vi "Read Serial Configs.vi"(8 "error in (no error)":errorcluster, 10 "Item Ref in":T2 format="%.0x", 11 "Refnum in":T1) -> (0 "error out":errorcluster, 2 "Item Ref out":T2 format="%.0x", 3 "Refnum out":T1)   [LabVIEW 2015, in "Modbus Master System Explorer.lvlib"]
uses:
  Modbus Master System Explorer.lvlib
  <vilib>/Utility/config.llb/Config Data RefNum.ctl
  <vilib>/NI Veristand/Custom Device API/Custom Device Item Ref.ctl
  Shared/Controls/Flow Control.ctl
  Shared/Controls/Serial Type.ctl
  Shared/Controls/Parity.ctl
  <vilib>/Utility/config.llb/Read Key (String).vi
  <vilib>/Utility/config.llb/Read Key (U32).vi
  <vilib>/Utility/config.llb/NI_LVConfig.lvlib
  Shared/Modbus Master Shared.lvlib
  <vilib>/NI VeriStand/Custom Device API/Custom Device API.lvlib
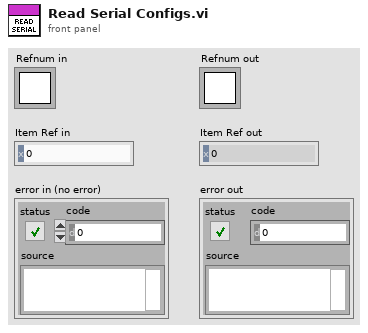
[diagram p1: front panel]
types:
  T1 = typedef "NI_LVConfig.lvlib/Config Data RefNum.ctl" = refnum<k1>
  T2 = typedef "Custom Device API.lvlib/Custom Device Item Ref.ctl" = u64
  T3 = typedef "Modbus Master Shared.lvlib/Serial Type.ctl" = enum16{"RTU", "ASCII"}
  T4 = typedef "Modbus Master Shared.lvlib/Parity.ctl" = u16
  T5 = typedef "Modbus Master Shared.lvlib/Flow Control.ctl" = u16
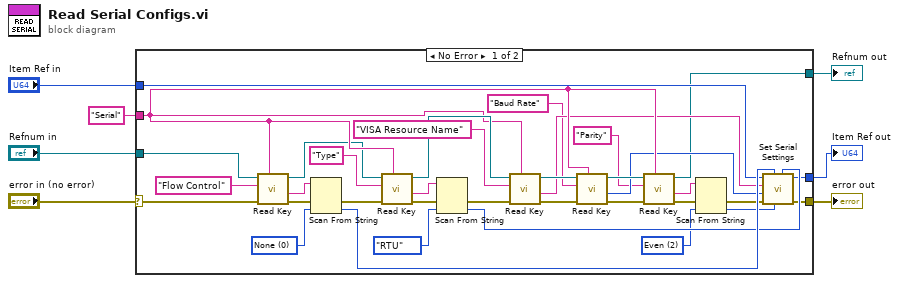
[diagram p0: block diagram]
diagram:
  n1 = case shown="No Error" "error in (no error)" {
    selector: "error in (no error)" -> [w36 w44]
    tunnel: "Refnum in" -> [w42 w43]
    tunnel: "Serial" ("section") -> [w40 _]
    tunnel: [w11 w44] -> w4
    tunnel: [w10 w45] -> w3
    tunnel: "Item Ref in" -> [w9 w45]
    tunnel: [w8 w43] -> w1
    frame No Error {
      w16 = T4 2 items=["None", "Odd", "Even", "Mark", "Space"] ("parity (even)")
      w32 = T5 0 items=["None", "XON/XOFF", "RTS/CTS", "XON/XOFF & RTS/CTS", "DTR/DSR", "XON/XOFF & DTR/DSR"] ("flow control (none)")
      n2 = call-poly <vilib>:"Read Key.vi"("section"=w40, "error in (no error)"=w36, "key"="Flow Control", "refnum"=w42) -> ("error out"=w29:errorcluster, "value"=w31:string, "refnum out"=w37:T1)  [unwired: 4 in, 1 out]
      n3 = Scan From String(input string=w31, error in=w29, default 1=w32) -> (error out=w28:errorcluster, output 1=w30:T5)  [unwired: 2 in, 2 out]
      n4 = call-poly <vilib>:"Read Key.vi"("section"=w40, "error in (no error)"=w28, "key"="Type", "refnum"=w37) -> ("error out"=w23:errorcluster, "value"=w27:string, "refnum out"=w41:T1)  [unwired: 4 in, 1 out]
      n5 = Scan From String(input string=w27, error in=w23, default 1=Serial_Type."RTU" ("serial type")) -> (error out=w22:errorcluster, output 1=w24:T3)  [unwired: 2 in, 2 out]
      n6 = call-poly <vilib>:"Read Key.vi"("section"=w40, "error in (no error)"=w22, "key"="VISA Resource Name", "refnum"=w41) -> ("error out"=w35:errorcluster, "value"=w20:string, "refnum out"=w39:T1)  [unwired: 4 in, 1 out]
      n7 = call-poly <vilib>:"Read Key.vi"("section"=w40, "error in (no error)"=w35, "key"="Baud Rate", "refnum"=w39) -> ("error out"=w34:errorcluster, "value"=w18:u32, "refnum out"=w38:T1)  [unwired: 4 in, 1 out]
      n8 = call-poly <vilib>:"Read Key.vi"("section"=w40, "error in (no error)"=w34, "key"="Parity", "refnum"=w38) -> ("error out"=w13:errorcluster, "value"=w15:string, "refnum out"=w8:T1)  [unwired: 4 in, 1 out]
      n9 = Scan From String(input string=w15, error in=w13, default 1=w16) -> (error out=w12:errorcluster, output 1=w14:T4)  [unwired: 2 in, 2 out]
      n10 = call "Set Serial Settings.vi"("serial type"=w24, "parity (even)"=w14, "flow control (none)"=w30, "error in (no error)"=w12, "baud rate"=w18, "VISA resource name"=w20, "Item Ref in"=w9) -> ("error out"=w11:errorcluster, "Item Ref out"=w10:T2)  [unwired: 3 in]
    }
    frame Error {
    }
  }
  "error out" <- w4
  "Item Ref out" <- w3
  "Refnum out" <- w1
